vi "Add Text Token.vi"(8 "Error In":errorcluster, 11 "Lexer In":refnum<class "Lexer.lvclass">) -> (0 "Error Out":errorcluster, 3 "Lexer Out":refnum<class "Lexer.lvclass">)   [LabVIEW 2018, in "Toolkit.lvlib" / "Lexer.lvclass"]
uses:
  Lexer.lvclass
  Lexer.lvclass/Lexer.ctl
  Tokens/Text/Text.lvclass
  D:/Users/cfield/Code/Field R&D Services/Mustache/trunk/src/Toolkit/Low-Level/Tokens/Abstract/Abstract.lvclass
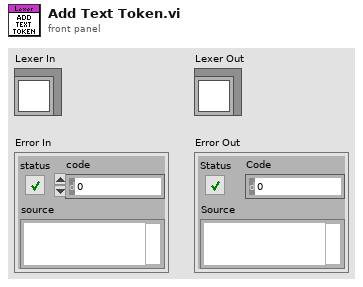
[diagram p1: front panel]
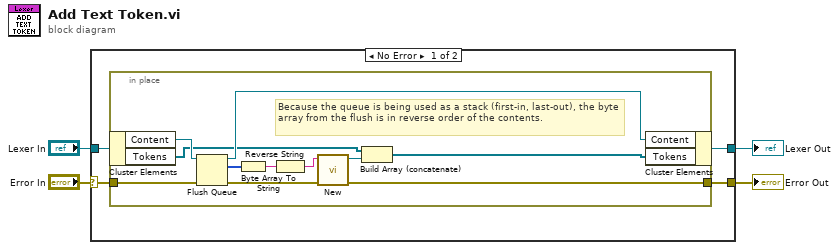
[diagram p0: block diagram]
diagram:
  n1 = case shown="No Error" "Error In" {
    selector: "Error In" -> [w6 w20]
    tunnel: [w5 w20] -> w4
    tunnel: [w8 w21] -> w3
    tunnel: "Lexer In" -> [w7 w21]
    frame No Error {
      n2 = in-place {
        in-place-border: w6 -> [w13]
        in-place-border: [w9] -> w5
        # "Because the queue is being used as a stack (first-in, last-out), the byte array from the flush is in reverse order of the contents."
        n3 = in-place-cluster #1(w7) -> ("Content"=w19:refnum<queue>, "Tokens"=w16:refnum<class "Abstract.lvclass">[])
        n4 = Flush Queue(queue=w19, error in (no error)=w13) -> (queue out=w18:refnum<queue>, remaining elements=w17:u8[], error out=w10:errorcluster)
        n5 = Byte Array To String(unsigned byte array=w17) -> (string=w12:string)
        n6 = Reverse String(1:w12) -> (0:w11:string)
        n7 = call "New.vi"("Error In"=w10, "Content"=w11) -> ("Error Out"=w9:errorcluster, "Text"=w15:refnum<class "Text.lvclass">)  [unwired: 8 in]
        n8 = Build Array (concatenate)(w16, w15) -> (w14:refnum<class "Abstract.lvclass">[])
        n9 = in-place-cluster #1("Content"=w18, "Tokens"=w14) -> (w8:refnum<class "Lexer.lvclass">)
      }
    }
    frame Error {
    }
  }
  "Error Out" <- w4
  "Lexer Out" <- w3
